vi "initialize Session Data.vi"(0 "OBJ - Session in":refnum<class "Serial Session.lvclass">, 11 "error in":errorcluster) -> (4 "OBJ - Session out":refnum<class "Serial Session.lvclass">, 15 "error out":errorcluster)   [LabVIEW 2015, in "Serial Session.lvclass"]
doc: "OVERRIDE VI\nPlaceholder for decendant sessions to initialize and set their default values"
uses:
  Serial Session.lvclass
  File Access/Config Data/Config Data.lvclass
  Typedefs/Serial Config.ctl
  Typedefs/Msg Config.ctl
  File Access/Config Data/Config Data.lvclass/Config Data.ctl
  File Access/Config Data/Accessors/Read Ref.vi
  <vilib>/Utility/config.llb/Read Key (String).vi
  <userlib>/_Session Fwk/Session - Root.lvclass
  Text Communication/Text Device Session.lvclass
  <vilib>/Utility/config.llb/NI_LVConfig.lvlib
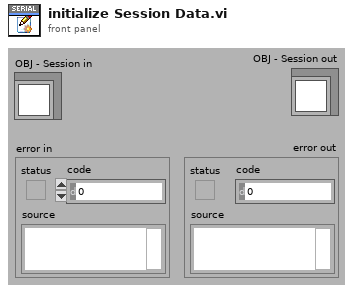
[diagram p1: front panel]
types:
  T1 = typedef "Session - Root.lvclass/Session Handle.ctl" = refnum<data-value>
  T2 = cluster{"EnTermChar":bool, "termChar":u8, "suppEnEnRd":bool, "sendEndEn":bool}
  T3 = typedef "Serial Session.lvclass/Msg Config.ctl" = cluster{"sendEndEn":bool, "suppEnEnRd":bool, "termChar":u8, "EnTermChar":bool}
  T4 = typedef "Serial Session.lvclass/Serial Config.ctl" = cluster{"baud rate":u32, "data bits":u16, "stop bits":u16, "parity":u16, "flow control":u16, "endModeforReads":u16, "endModeforWrites":u16}
  T5 = typedef "NI_LVConfig.lvlib/Config Data RefNum.ctl" = refnum<k1>
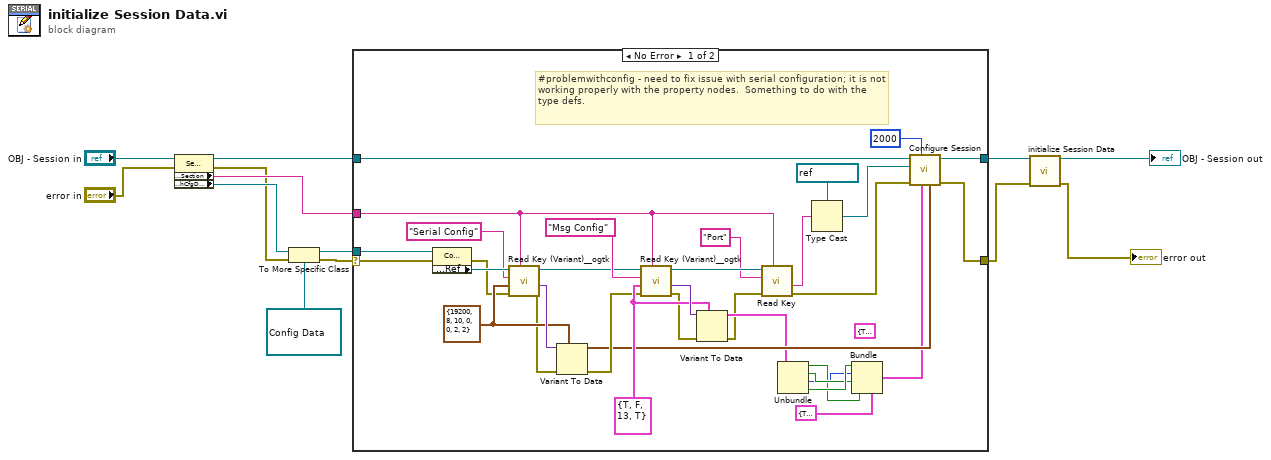
[diagram p0: block diagram]
diagram:
  n1 = property class="Serial Session"(reference="OBJ - Session in", error in="error in") -> (reference out=w11:refnum<class "Serial Session.lvclass">, error out=w5:errorcluster, "Accessors:Section"=w12:string, "Accessors:hCfgData"=w10:T1)
  n2 = To More Specific Class(target class=refnum<data-value> refnum ("hCfgData"), reference=w10, error in=w5) -> (specific class reference=w8:refnum<data-value>, error out=w7:errorcluster)
  n3 = case shown="No Error" w7 {
    selector: w7 -> [w34 w49]
    tunnel: [w26 w49] -> w2
    tunnel: [w29 w48] -> w4
    tunnel: w11 -> [w18 w48]
    tunnel: w8 -> [w47 _]
    tunnel: w12 -> [w36 _]
    frame No Error {
      (unwired) T2 {"EnTermChar"=TRUE, "termChar"=13, "suppEnEnRd"=FALSE, "sendEndEn"=TRUE} ("Message Cfg 2")
      w39 = T3 {"sendEndEn"=TRUE, "suppEnEnRd"=FALSE, "termChar"=13, "EnTermChar"=TRUE} ("Msg Configuration")
      w44 = T4 {"baud rate"=19200, "data bits"=8, "stop bits"=10, "parity"=0, "flow control"=0, "endModeforReads"=2, "endModeforWrites"=2} ("Serial Config")
      # "#problemwithconfig - need to fix issue with serial configuration; it is not working properly with the property nodes.  Something to do with the type defs."
      n4 = property class="Config Data"(reference=w47, error in=w34) -> (error out=w33:errorcluster, "Accessors:Ref"=w46:T5)  [unwired: 1 out]
      n5 = call <userlib>:"Read Key (Variant)__ogtk.vi"("section"=w36, "error in (no error)"=w33, "type"=w44, "key (optional)"="Serial Config", "refnum"=w46) -> ("error out"=w43:errorcluster, "key-value"=w45:variant, "refnum out"=w32:T5)  [unwired: 3 in, 1 out]
      n6 = Variant To Data(error in=w43, type=w44, Variant=w45) -> (data=w25:T4, error out=w38:errorcluster)
      n7 = call <userlib>:"Read Key (Variant)__ogtk.vi"("section"=w36, "error in (no error)"=w38, "type"=w39, "key (optional)"="Msg Config", "refnum"=w32) -> ("error out"=w15:errorcluster, "key-value"=w40:variant, "refnum out"=w37:T5)  [unwired: 3 in, 1 out]
      n8 = Variant To Data(error in=w15, type=w39, Variant=w40) -> (data=w24:T3, error out=w14:errorcluster)
      n9 = call-poly <vilib>:"Read Key.vi"("section"=w36, "error in (no error)"=w14, "key"="Port", "refnum"=w37) -> ("error out"=w28:errorcluster, "value"=w31:string)  [unwired: 4 in, 2 out]
      n10 = Unbundle(w24) -> ("sendEndEn"=w20:bool, "suppEnEnRd"=w21:bool, "termChar"=w19:u8, "EnTermChar"=w22:bool)
      n11 = Type Cast(type=refnum<visa-resource-name> "COM5" ("VISA Resource"), x=w31) -> (*(type *) &x=w27:refnum<visa-resource-name>)
      n12 = Bundle(cluster=T2 {"EnTermChar"=TRUE, "termChar"=13, "suppEnEnRd"=FALSE, "sendEndEn"=TRUE} ("Message Cfg 2"), "EnTermChar"=w22, "termChar"=w19, "suppEnEnRd"=w21, "sendEndEn"=w20) -> (w16:T2)
      n13 = call "Configure Session.vi"("serialCfg"=w25, "Message Cfg"=w16, "timeout"=u32 2000, "error in"=w28, "VISA Resource"=w27, "Serial Session"=w18) -> ("error out"=w26:errorcluster, "Serial Session out"=w29:refnum<class "Serial Session.lvclass">)  [unwired: 4 in]
    }
    frame Error {
    }
  }
  n14 = call-parent "initialize Session Data.vi"("OBJ - Session in"=w4, "error in"=w2) -> ("OBJ - Session out"=→"OBJ - Session out":refnum<class "Serial Session.lvclass">, "error out"=→"error out":errorcluster)  [unwired: 12 in]
